vi "Get Attributes From Ini File.vi"(8 "error in (no error)":errorcluster, 10 "section":string="ScriptsDialog", 11 "UIConfiguration in":refnum<class "UIConfiguration.lvclass">) -> (0 "error out":errorcluster, 3 "UIConfiguration out":refnum<class "UIConfiguration.lvclass">)   [LabVIEW 2015, in "UIConfiguration.lvclass"]
uses:
  UIConfiguration.lvclass
  UIConfiguration.lvclass/UIConfiguration.ctl
  <vilib>/Utility/config.llb/NI_LVConfig.lvlib
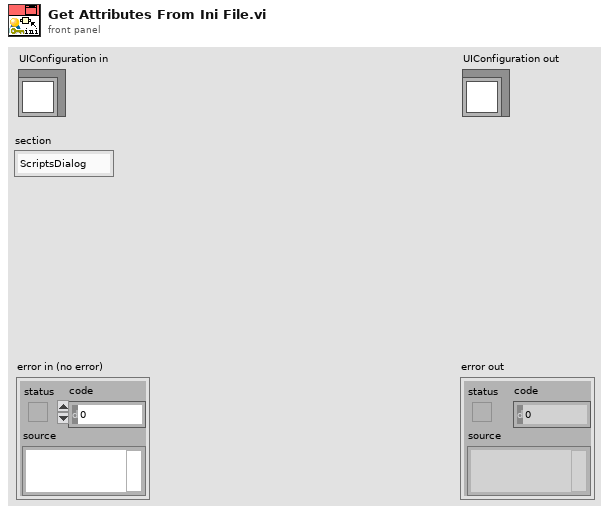
[diagram p1: front panel]
types:
  T1 = typedef "NI_LVConfig.lvlib/Config Data RefNum.ctl" = refnum<k1>
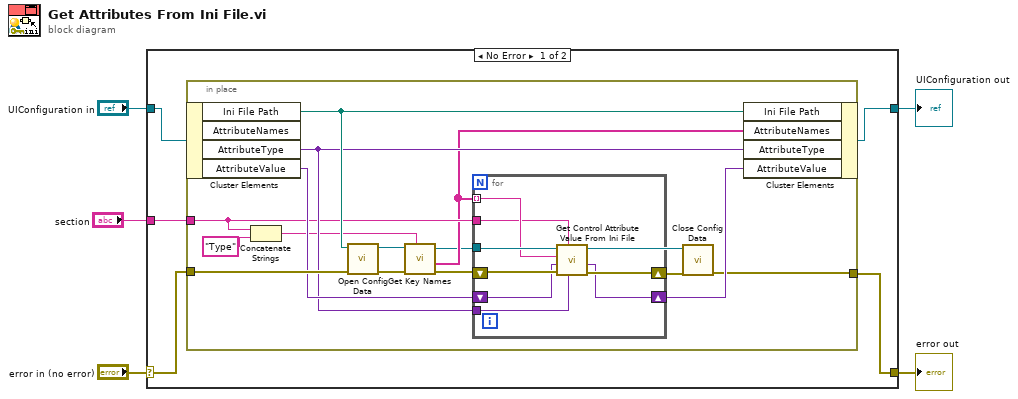
[diagram p0: block diagram]
diagram:
  n1 = case shown="No Error" "error in (no error)" {
    selector: "error in (no error)" -> [w8 w35]
    tunnel: [w6 w35] -> w4
    tunnel: [w7 w34] -> w2
    tunnel: "UIConfiguration in" -> [w10 w34]
    tunnel: "section" -> [w9 _]
    frame No Error {
      n2 = in-place {
        in-place-border: w9 -> [w18]
        in-place-border: w8 -> [w25]
        in-place-border: [w11] -> w6
        n3 = in-place-cluster #1(w10) -> ("Ini File Path"=w23:path, "AttributeType"=w22:variant, "AttributeValue"=w24:variant)  [unwired: 1 out]
        n4 = Concatenate Strings(w18, "Type" ("string")) -> (w16:string)
        n5 = call <vilib>:"Open Config Data.vi"("error in (no error)"=w25, "configuration file path"=w23) -> ("error out"=w19:errorcluster, "refnum"=w20:T1)  [unwired: 7 in, 1 out]
        n6 = call <vilib>:"Get Key Names.vi"("section"=w16, "error in (no error)"=w19, "refnum"=w20) -> ("error out"=w14:errorcluster, "key names"=w15:string[], "refnum out"=w12:T1)  [unwired: 5 in, 1 out]
        n7 = for {
          tunnel: w12 -> [w32]
          tunnel: w15 -> [w33] mode=indexing
          tunnel: w22 -> [w29]
          tunnel: w18 -> [w27]
          shift-right: [w26] -> w21
          shift-left: w24 -> [w28]
          shift-right: [w30] -> w13
          shift-left: w14 -> [w31]
          n8 = call "Get Control Attribute Value From Ini File.vi"("AttributeType"=w29, "Section Name"=w27, "error in (no error)"=w31, "AttributeValue"=w28, "AttributeNames"=w33, "Ini Config Ref"=w32) -> ("error out"=w30:errorcluster, "AttributeValue Out"=w26:variant)  [unwired: 2 in, 2 out]
        }
        n9 = call <vilib>:"Close Config Data.vi"("error in (no error)"=w13, "refnum"=w12) -> ("error out"=w11:errorcluster)  [unwired: 8 in, 1 out]
        n10 = in-place-cluster #1("Ini File Path"=w23, "AttributeNames"=w15, "AttributeType"=w22, "AttributeValue"=w21) -> (w7:refnum<class "UIConfiguration.lvclass">)
      }
    }
    frame Error {
    }
  }
  "error out" <- w4
  "UIConfiguration out" <- w2
